vi "Parameterized Data to JSON.vi"(10 "Outputs":map{string, variant}(c390), 11 "Inputs":map{string, variant}(c390)) -> (3 "<JSON>":string)   [LabVIEW 2020, in "Approval Tests.lvlib"]
uses:
  Approval Tests.lvlib
  <vilib>/PNR/JSONtext Object Serialization/Generic Object Serializer/Generic Object Serializer.lvclass
  C:/Program Files/National Instruments/LabVIEW 2026/vi.lib/JDP Science/JSONtext/LVClass Serializer/JSONtext LVClass Serializer.lvclass
  28634094-913e-473c-8292-0b8dd8e8d3ae.vi
  9220d738-47a7-4d64-8b80-0b8da982d701.vi
  <vilib>/JDP Science/JSONtext/Variant to JSON Text.vi
  <vilib>/JDP Science/JSONtext/support/Format JSON Object.vi
  <vilib>/JDP Science/JSONtext/JSONtext.lvlib
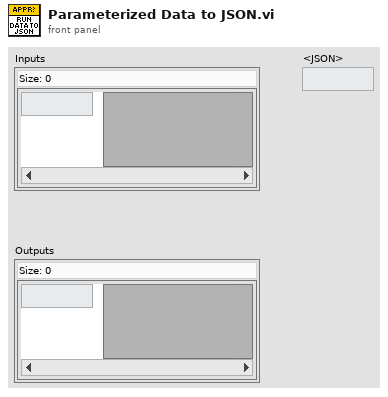
[diagram p1: front panel]
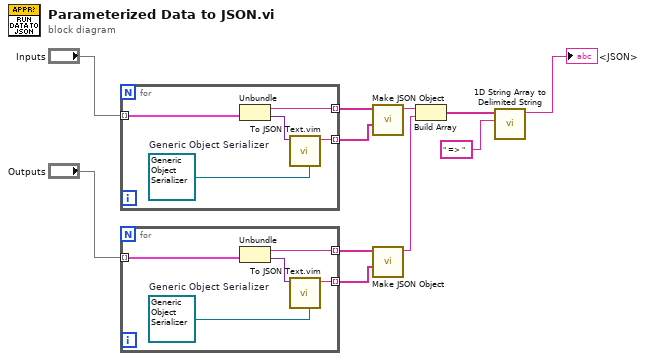
[diagram p0: block diagram]
diagram:
  n1 = for {
    tunnel: "Inputs" -> [w16] mode=indexing
    tunnel: [w14] -> w8 mode=indexing
    tunnel: [w13] -> w9 mode=indexing
    w12 = refnum<class "Generic Object Serializer.lvclass"> refnum  # Generic Object Serializer
    n2 = Unbundle(w16) -> ("key"=w14:string, "Variant"=w15:variant)
    n3 = call "To JSON Text.vim"("LVClass Serializer"=w12, "Anything"=w15) -> ("<JSON>"=w13:string)  [unwired: 8 in, 1 out]
  }
  n4 = for {
    tunnel: "Outputs" -> [w21] mode=indexing
    tunnel: [w19] -> w5 mode=indexing
    tunnel: [w18] -> w4 mode=indexing
    w17 = refnum<class "Generic Object Serializer.lvclass"> refnum  # Generic Object Serializer
    n5 = Unbundle(w21) -> (w19:string, "Value"=w20:variant)
    n6 = call "To JSON Text.vim"("LVClass Serializer"=w17, "Anything"=w20) -> ("<JSON>"=w18:string)  [unwired: 8 in, 1 out]
  }
  n7 = call <vilib>:"Make JSON Object.vi"("JSON Items"=w9, "Item Names"=w8) -> ("<JSON>"=w10:string)  [unwired: 8 in, 1 out]
  n8 = call <vilib>:"Make JSON Object.vi"("JSON Items"=w4, "Item Names"=w5) -> ("<JSON>"=w11:string)  [unwired: 8 in, 1 out]
  n9 = Build Array(w10, w11) -> (w3:string[])
  n10 = call <vilib>:"1D String Array to Delimited String.vi"("delimiter"=" => ", "string array"=w3) -> ("delimited string"=→"<JSON>":string)  [unwired: 9 in]
